vi "Define_ModeFunction.vi"(8 "error in (no error)":errorcluster, 10 "SMU Config":T1, 11 "VISA Refnum in":refnum<visa-resource-name>) -> (0 "error out":errorcluster, 3 "VISA Refnum out":refnum<visa-resource-name>)   [LabVIEW 2012]
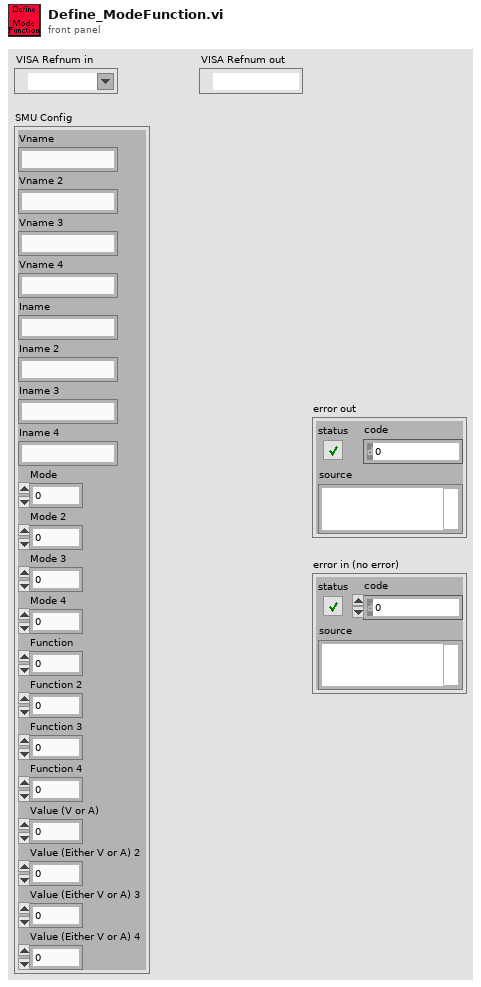
[diagram p1: front panel]
types:
  T1 = cluster{"Vname":string, "Vname 2":string, "Vname 3":string, "Vname 4":string, "Iname":string, "Iname 2":string, "Iname 3":string, "Iname 4":string, "Mode":u16, "Mode 2":u16, "Mode 3":u16, "Mode 4":u16, "Function":u16, "Function 2":u16, "Function 3":u16, "Function 4":u16, "Value (V or A)":dbl, "Value (Either V or A) 2":dbl, "Value (Either V or A) 3":dbl, "Value (Either V or A) 4":dbl}
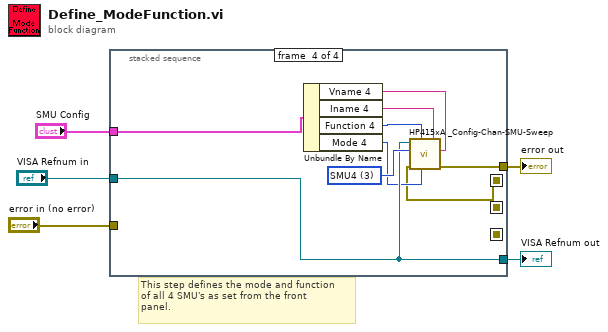
[diagram p0: block diagram]
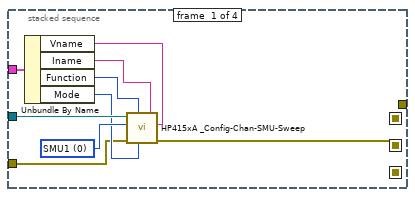
[diagram p2: hidden frame]
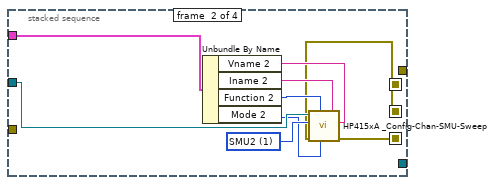
[diagram p3: hidden frame]
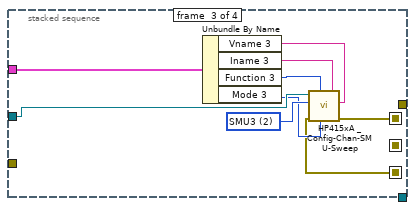
[diagram p4: hidden frame]
diagram:
  # "This step defines the mode and function\nof all 4 SMU's as set from the front\npanel."
  n1 = stacked-sequence {
    seq-local: [w6 _ _ _] -> [_ w16 _ _]
    seq-local: [_ w15 _ _] -> [_ _ w25 _]
    seq-local: [_ _ w24 _] -> [_ _ _ w34]
    tunnel: "VISA Refnum in" -> [w13 w22 w31 w40]
    tunnel: [_ _ _ w40] -> w5
    tunnel: "SMU Config" -> [w9 w17 w30 w39]
    tunnel: "error in (no error)" -> [w7 _ _ _]
    tunnel: [_ _ _ w33] -> w4
    frame #0 {
      w14 = u32 0 items=["SMU1  ", "SMU2  ", "SMU3  ", "SMU4  ", "SMU5  ", "SMU6  "] ("unit to configure")
      n2 = Unbundle By Name(w9) -> ("Vname"=w8:string, "Iname"=w10:string, "Function"=w11:u16, "Mode"=w12:u16)
      n3 = call "HP415xA _Config-Chan-SMU-Sweep.vi"("V name (max 6 chars)"=w8, "I name (max 6 chars)"=w10, "mode"=w12, "function"=w11, "error in (no error)"=w7, "unit to configure"=w14, "VISA session"=w13) -> ("error out"=w6:errorcluster)  [unwired: 2 in]
    }
    frame #1 {
      w23 = u32 1 items=["SMU1  ", "SMU2  ", "SMU3  ", "SMU4  ", "SMU5  ", "SMU6  "] ("unit to configure")
      n4 = Unbundle By Name(w17) -> ("Vname 2"=w21:string, "Iname 2"=w20:string, "Function 2"=w19:u16, "Mode 2"=w18:u16)
      n5 = call "HP415xA _Config-Chan-SMU-Sweep.vi"("V name (max 6 chars)"=w21, "I name (max 6 chars)"=w20, "mode"=w18, "function"=w19, "error in (no error)"=w16, "unit to configure"=w23, "VISA session"=w22) -> ("error out"=w15:errorcluster)  [unwired: 2 in]
    }
    frame #2 {
      w32 = u32 2 items=["SMU1  ", "SMU2  ", "SMU3  ", "SMU4  ", "SMU5  ", "SMU6  "] ("unit to configure")
      n6 = Unbundle By Name(w30) -> ("Vname 3"=w29:string, "Iname 3"=w28:string, "Function 3"=w27:u16, "Mode 3"=w26:u16)
      n7 = call "HP415xA _Config-Chan-SMU-Sweep.vi"("V name (max 6 chars)"=w29, "I name (max 6 chars)"=w28, "mode"=w26, "function"=w27, "error in (no error)"=w25, "unit to configure"=w32, "VISA session"=w31) -> ("error out"=w24:errorcluster)  [unwired: 2 in]
    }
    frame #3 {
      w41 = u32 3 items=["SMU1  ", "SMU2  ", "SMU3  ", "SMU4  ", "SMU5  ", "SMU6  "] ("unit to configure")
      n8 = Unbundle By Name(w39) -> ("Vname 4"=w38:string, "Iname 4"=w37:string, "Function 4"=w36:u16, "Mode 4"=w35:u16)
      n9 = call "HP415xA _Config-Chan-SMU-Sweep.vi"("V name (max 6 chars)"=w38, "I name (max 6 chars)"=w37, "mode"=w35, "function"=w36, "error in (no error)"=w34, "unit to configure"=w41, "VISA session"=w40) -> ("error out"=w33:errorcluster)  [unwired: 2 in]
    }
  }
  "VISA Refnum out" <- w5
  "error out" <- w4
